vi "DPOAE I-O.vi"(0 "State in":T4) -> (4 "State out":T4)   [LabVIEW 2020]
uses:
  CFTS VIs/CFTS-Experiment State.ctl
  Typedefs/DP-Queue Data.ctl
  Typedefs/DP-Parameters.ctl
  Typedefs/DP-Stimulus Params.ctl
  Typedefs/DP-Response Params.ctl
  epl-vi-lib/Utility VIs/File IO VIs/Configuration File Wrapper VIs/Config-Write Key (string).vi
panel:
  in  "Probe Mic Gain (dB)":dbl
  in  "Save raw data?":bool=TRUE
  out "User":string
  out "Run #":u16=14
  out "ID #":u16=1
  in  "Avg specs":T1={"# Time avgs "=8, "# Spectrum avgs"=4}
  in  "Stimulus":T2={"Ear"=enum."Right", "f2 freqs (kHz)"="5.6;8.0;11.3;16;22.6;32;", "Start (dB)"=20.0, "Stop (dB)"=70.0, "Step (dB)"=10.0, "Mode"=enum."L1 = L2 + 10 dB"}
  out "result":T3
  out "Path":path
  in  "Start":bool
  in  "Stop":bool
  out "Error":bool
  out "Freqs":cluster{"f1":dbl, "f2":dbl, "2f1-f2":dbl}={"f1"=9419.759114583332, "f2"=11291.50390625, "2f1-f2"=7548.014322916664} {"2f1-f2" format="%.3f"; "f1" format="%.3f"; "f2" format="%.3f"}
  out "DP window":cluster{i32, "df (Hz)":dbl, dbl[]}(graph)={0, "df (Hz)"=0.02, []}
  out "I-O Plot":cluster{cluster{dbl, dbl}[]}[](graph)
  in  "Notes":string
  out "Full Spectrum":cluster{i32, "Freq Resolution":dbl, dbl[]}(graph)={0, "Freq Resolution"=20.345052083333332, []}
  in  "RETURN":bool
  # "Stimulus"
  # "Averaging"
  # "Response"
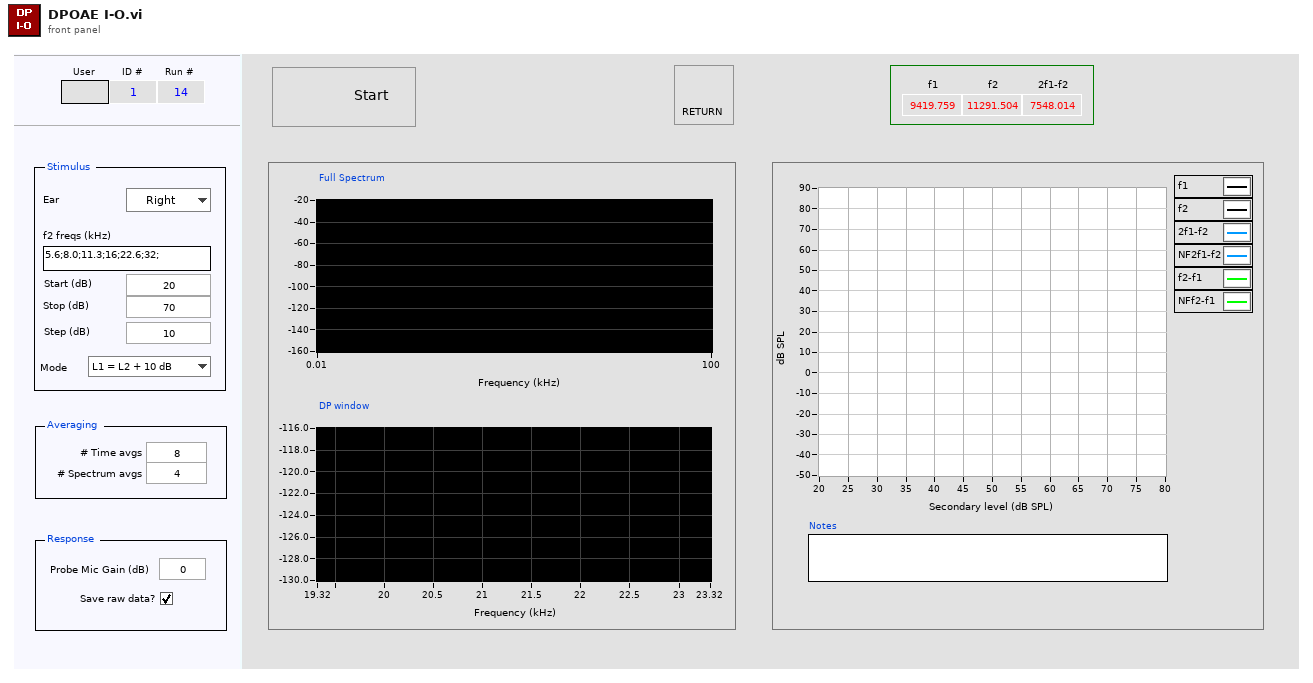
[diagram p1: front panel]
types:
  T1 = cluster{"# Time avgs ":i32, "# Spectrum avgs":i32}
  T2 = cluster{"Ear":enum16{"Right", "Left"}, "f2 freqs (kHz)":string, "Start (dB)":dbl, "Stop (dB)":dbl, "Step (dB)":dbl, "Mode":enum16{"L1 = L2", "L1 = L2 + 10 dB"}}
  T3 = cluster{"file":path, "aborted":bool, "error":errorcluster}
  T4 = typedef "CFTS-Experiment State.ctl" = cluster{"Experimenter":string, "Number":u32, "Right":string, "Left":string, "Data Folder":path, "Version":string, "End Exposure Time":dbl, "Exposure Duration":string, "Run #":cluster{"CAP":i32, "ABR":i32, "DP":i32, "VsEP":i32, "SFOAE":i32}}
  T5 = typedef "DP-Queue Data.ctl" = cluster{"action":string, "path":path, "Acoustic system":string, "Parameters":T6}
  T6 = typedef "DP-Parameters.ctl" = cluster{"Stimulus":T7, "Response":T8}
  T7 = typedef "DP-Stimulus Params.ctl" = cluster{"Ear":enum16{"Right", "Left"}, "f2 freqs (kHz)":string, "Start (dB)":dbl, "Stop (dB)":dbl, "Step (dB)":dbl, "Mode":enum16{"L1 = L2", "L1 = L2 + 10 dB"}, "override recal":bool, "Sampling Rate (Hz)":dbl, "Frame (ms)":dbl}
  T8 = typedef "DP-Response Params.ctl" = cluster{"Time avgs":i32, "Freq avgs":i32, "Mic gain (dB)":dbl, "Save raw":bool}
  T9 = enum8{"Enabled", "Disabled", "Disabled and Grayed Out"}
  T10 = typedef "DP-Runtime State.ctl" = cluster{"#spectra avgs":i32[], "#time avgs":i32[], "dt (ms)":dbl, "df (kHz)":dbl, "pts/frame":i32, "Save raw?":bool, "Data File":path, "Sampling rate (Hz)":dbl, "Probe Tube Sensitivity":cluster{"Frequency":dbl[], "Mag":dbl[], "Phase":dbl[]}, "Mic gain (dB)":dbl, "frames/buffer":i32, "pts/buffer":i32, "speakers":string[], "mic":string}
  T11 = typedef "DP-Freqs.ctl" = cluster{"f1":dbl, "f2":dbl, "2f1-f2":dbl}
  T12 = typedef "DP-Level Series Info.ctl" = cluster{"freq":dbl[], "atten":dbl[][], "ntime":i32[], "nfreq":i32[], "raw file":path, "flip":bool}
  T13 = cluster{"Data File":path, "aborted":bool, "error out":errorcluster}
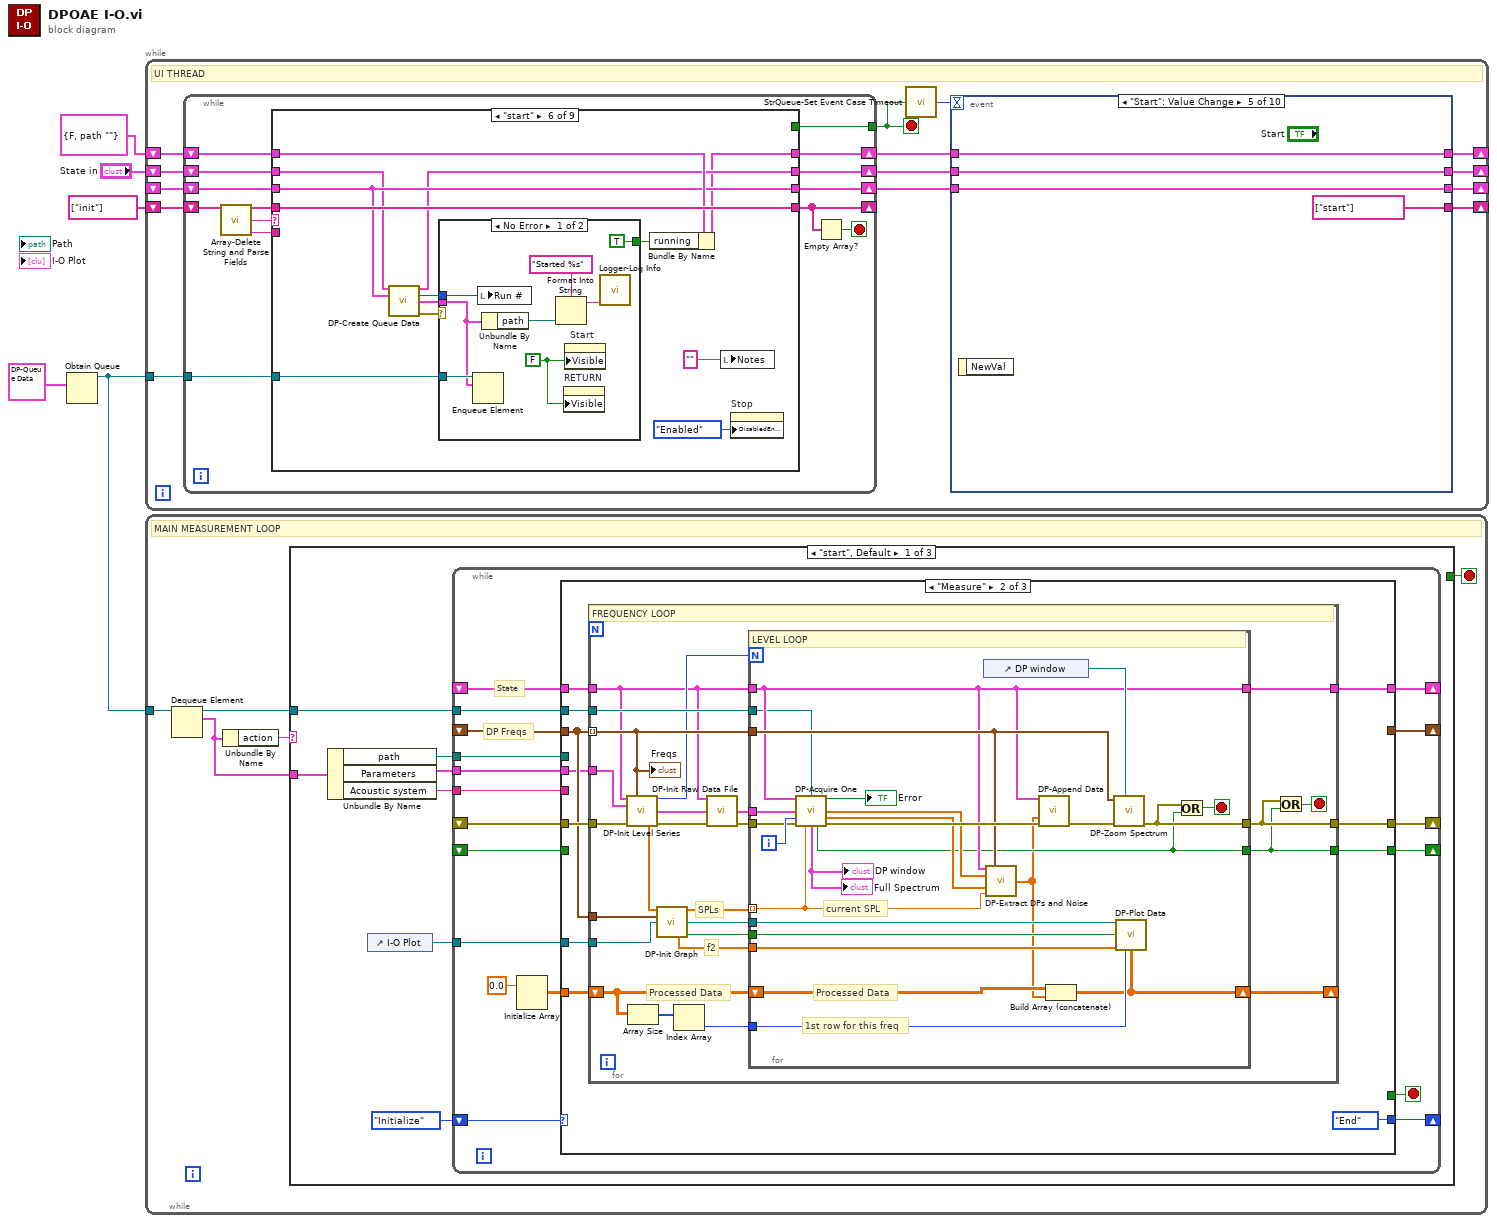
[diagram p0: block diagram]
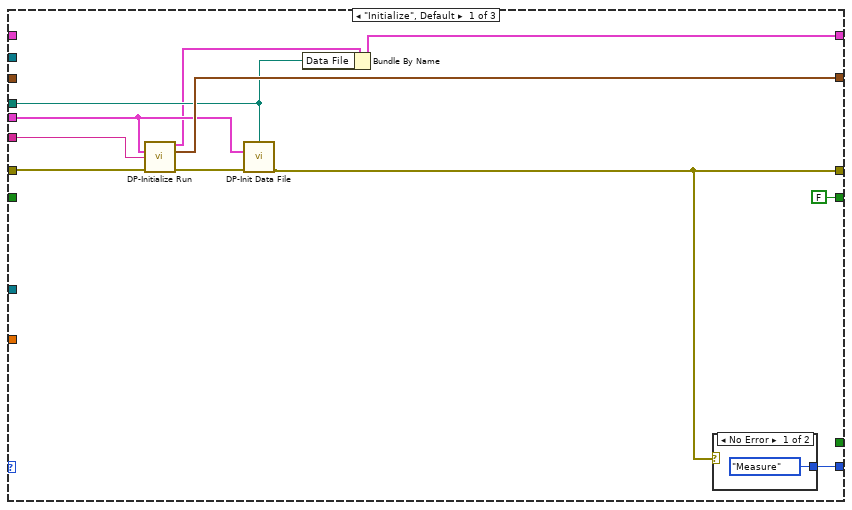
[diagram p2: hidden frame]
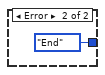
[diagram p3: hidden frame]
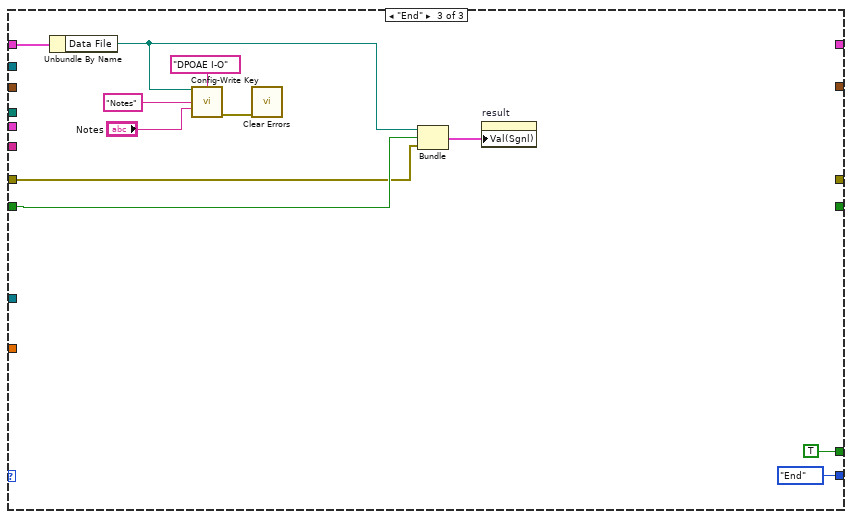
[diagram p4: hidden frame]
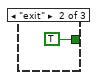
[diagram p5: hidden frame]
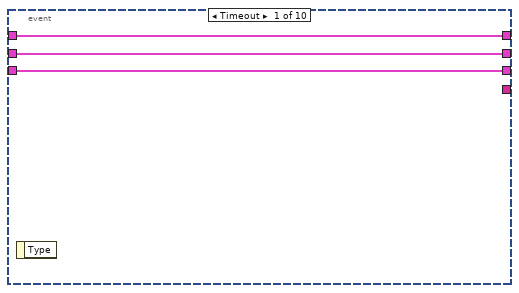
[diagram p7: hidden frame]
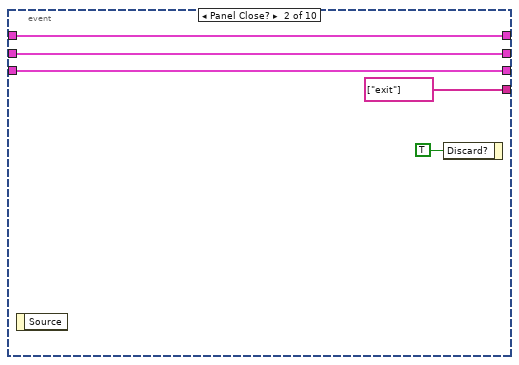
[diagram p8: hidden frame]
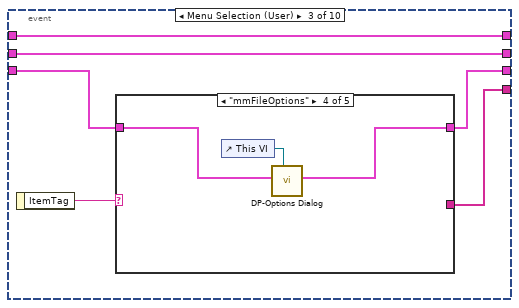
[diagram p9: hidden frame]
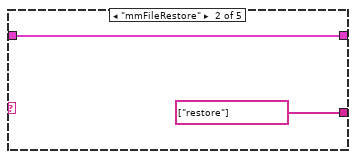
[diagram p11: hidden frame]
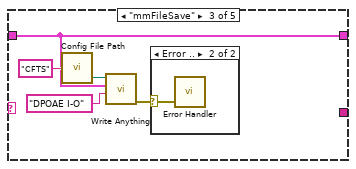
[diagram p12: hidden frame]
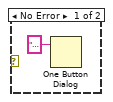
[diagram p13: hidden frame]
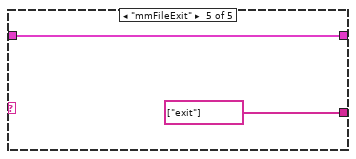
[diagram p14: hidden frame]
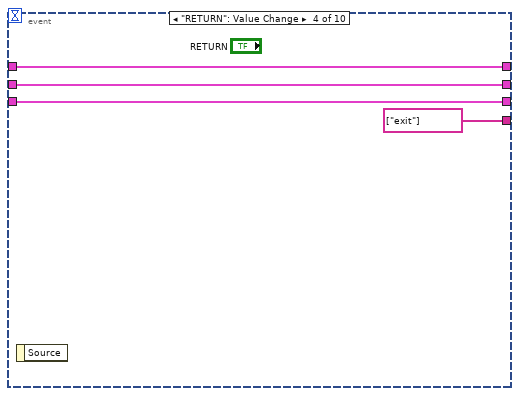
[diagram p15: hidden frame]
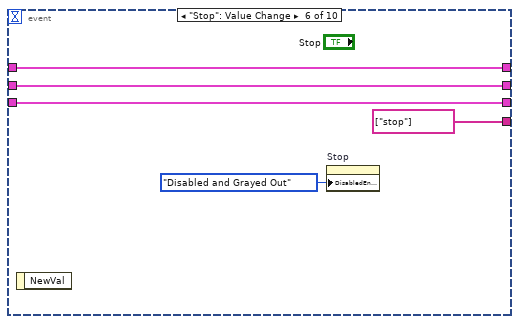
[diagram p16: hidden frame]
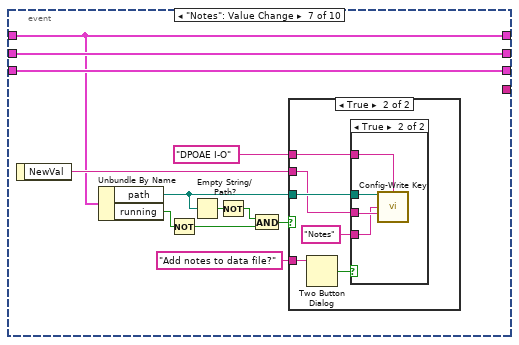
[diagram p17: hidden frame]
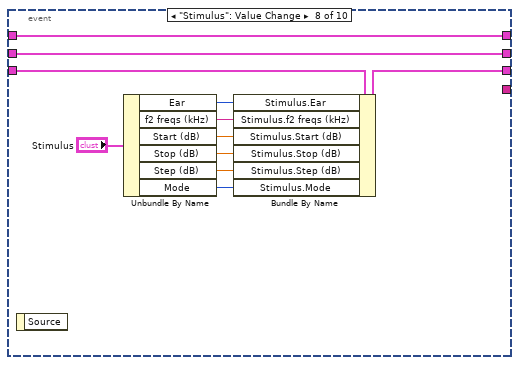
[diagram p20: hidden frame]
diagram:
  n1 = Obtain Queue(element data type=T5 {"action"="", "path"=path "", "Acoustic system"="", "Parameters"={"Stimulus"={"Ear"=enum."Right", "f2 freqs (kHz)"="", "Start (dB)"=0.0, "Stop (dB)"=0.0, "Step (dB)"=0.0, "Mode"=enum."L1 = L2", "override recal"=FALSE, "Sampling Rate (Hz)"=0.0, "Frame (ms)"=0.0}, "Response"={"Time avgs"=0, "Freq avgs"=0, "Mic gain (dB)"=0.0, "Save raw"=FALSE}}} ("data")) -> (queue out=w2:refnum<queue>)  [unwired: 4 in, 2 out]
  n2 = while {
    tunnel: w2 -> [w16]
    shift-right: [w14] -> _
    shift-left: string[] ["init"] -> [w15]
    shift-right: [w12] -> _
    shift-left: cluster{"running":bool, "path":path} {"running"=FALSE, "path"=path ""} -> [w13]
    shift-right: [w10] -> _
    shift-left: "State in" -> [w17]
    shift-right: [w8] -> _
    shift-left: _ -> [w6]
    stop <- w18 stop-if-true
    # "UI THREAD"
    n3 = while {
      shift-right: [w146] -> _
      shift-left: w15 -> [w143]
      tunnel: [w144] -> w18
      tunnel: w16 -> [w139]
      shift-right: [w137] -> w11
      shift-left: w13 -> [w138]
      shift-right: [w136] -> w9
      shift-left: w17 -> [w140]
      shift-right: [w135] -> w7
      shift-left: w6 -> [w134]
      stop <- w145 stop-if-true
      n4 = call "Array-Delete String and Parse Fields.vi"("Array in"=w143) -> ("Array out"=w142:string[], "Field 1"=w141:string, "Field 2"=w133:string)  [unwired: 10 in, 2 out]
      n5 = case shown="\"start\"" w141 {
        tunnel: w142 -> [w150 w159 _ w174 w192 w205 w223 w226 w257]
        tunnel: [w150 w159 string[] ["restore"] ("Array out") w170 w192 w205 w223 w225 w257] -> w146
        tunnel: [_ TRUE _ _ _ _ _ _ _] -> w144
        tunnel: w140 -> [w148 w156 w165 w172 w190 w197 w221 w229 w254]
        tunnel: w139 -> [_ w152 _ _ _ w201 w216 _ _]
        tunnel: w138 -> [w149 w157 w163 w173 w191 w202 w222 w230 w256]
        tunnel: [w149 w157 w163 w173 w191 w194 w222 w230 w256] -> w137
        tunnel: [w148 w156 w165 w172 w190 w196 w221 w224 w254] -> w136
        tunnel: [w147 w155 w161 w171 w181 w198 w220 w235 w255] -> w135
        tunnel: w134 -> [w147 w155 w161 _ w181 w198 w220 w235 w255]
        tunnel: w133 -> [_ _ _ _ _ _ _ w227 _]
        frame "", Default {
        }
        frame "exit" {
          n6 = Bundle By Name(cluster=T5 {"action"="", "path"=path "", "Acoustic system"="", "Parameters"={"Stimulus"={"Ear"=enum."Right", "f2 freqs (kHz)"="", "Start (dB)"=0.0, "Stop (dB)"=0.0, "Step (dB)"=0.0, "Mode"=enum."L1 = L2", "override recal"=FALSE, "Sampling Rate (Hz)"=0.0, "Frame (ms)"=0.0}, "Response"={"Time avgs"=0, "Freq avgs"=0, "Mic gain (dB)"=0.0, "Save raw"=FALSE}}} ("data"), "action"="exit") -> (w151:T5)
          n7 = Enqueue Element(queue=w152, element=w151) -> ()  [unwired: 2 in, 3 out]
          "State out" <- w156
        }
        frame "init" {
          w164 = TRUE
          n8 = Unbundle By Name(w165) -> ("Experimenter"=→"User":string, "Number"=→"ID #":u32, "Run #.DP"=→"Run #":i32)
          n9 = property on="RETURN" class="Bool"("Visible"=w164) -> ()  [unwired: 2 in, 2 out]
          n10 = property on="Start" class="Bool"("Visible"=w164) -> ()  [unwired: 2 in, 2 out]
          n11 = local write "Error"(FALSE ("Error")) -> ()
        }
        frame "restore" {
          n12 = call "DP-Restore Defaults.vi"() -> ("Parameters"=w171:T6)  [unwired: 14 in, 1 out]
          n13 = Build Array (concatenate)(w174, "show params") -> (w170:string[])
        }
        frame "show params" {
          n14 = Unbundle By Name(w181) -> ("Stimulus.Ear"=w188:enum16{"Right", "Left"}, "Stimulus.f2 freqs (kHz)"=w187:string, "Stimulus.Start (dB)"=w186:dbl, "Stimulus.Stop (dB)"=w185:dbl, "Stimulus.Step (dB)"=w184:dbl, "Stimulus.Mode"=w183:enum16{"L1 = L2", "L1 = L2 + 10 dB"})
          n15 = Unbundle By Name(w181) -> ("Response.Time avgs"=w179:i32, "Response.Freq avgs"=w178:i32, "Response.Mic gain (dB)"=w176:dbl, "Response.Save raw"=w175:bool)
          n16 = local read "Stimulus"() -> (w189:T2)
          n17 = local write "Probe Mic Gain (dB)"(w176) -> ()
          n18 = local write "Save raw data?"(w175) -> ()
          n19 = Bundle By Name(cluster=w189, "Ear"=w188, "f2 freqs (kHz)"=w187, "Start (dB)"=w186, "Stop (dB)"=w185, "Step (dB)"=w184, "Mode"=w183) -> (w182:T2)
          n20 = local read "Avg specs"() -> (w180:T1)
          n21 = Bundle By Name(cluster=w180, "# Time avgs"=w179, "# Spectrum avgs"=w178) -> (w177:T1)
          n22 = local write "Stimulus"(w182) -> ()
          n23 = local write "Avg specs"(w177) -> ()
        }
        frame "start" {
          n24 = call "DP-Create Queue Data.vi"("State in"=w197, "Parameters"=w198) -> ("State out"=w196:T4, "run"=w195:i32, "data"=w200:T5, "error out"=w199:errorcluster)  [unwired: 10 in]
          n25 = case shown="No Error" w199 {
            selector: w199 -> [_ w215]
            tunnel: w201 -> [w213 _]
            tunnel: w200 -> [w209 _]
            tunnel: w195 -> [w211 _]
            tunnel: [TRUE _] -> w193
            frame No Error {
              w212 = FALSE
              n26 = Enqueue Element(queue=w213, element=w209) -> ()  [unwired: 2 in, 3 out]
              n27 = local write "Run #"(w211) -> ()
              n28 = Unbundle By Name(w209) -> ("path"=w208:path)
              n29 = Format Into String(format string="Started %s", w208) -> (resulting string=w206:string)  [unwired: 2 in, 1 out]
              n30 = property on="RETURN" class="Bool"("Visible"=w212) -> ()  [unwired: 2 in, 2 out]
              n31 = property on="Start" class="Bool"("Visible"=w212) -> ()  [unwired: 2 in, 2 out]
              n32 = call "Logger-Log Info.vi"("Message"=w206) -> ()  [unwired: 14 in, 1 out]
            }
            frame Error {
              n33 = call "Logger-Check and Log Error.vi"("error in (no error)"=w215) -> ("error out"=w214:errorcluster)  [unwired: 14 in]
              n34 = call "Error Handler.vi"("error in (no error)"=w214) -> ()  [unwired: 12 in, 3 out]
            }
          }
          n35 = Bundle By Name(cluster=w202, "running"=w193) -> (w194:cluster{"running":bool, "path":path})
          n36 = local write "Notes"("" ("Notes")) -> ()
          n37 = property on="Stop" class="Bool"("DisabledEnum"=T9."Enabled" ("Disabled")) -> ()  [unwired: 2 in, 2 out]
        }
        frame "stop" {
          n38 = Bundle By Name(cluster=T5 {"action"="", "path"=path "", "Acoustic system"="", "Parameters"={"Stimulus"={"Ear"=enum."Right", "f2 freqs (kHz)"="", "Start (dB)"=0.0, "Stop (dB)"=0.0, "Step (dB)"=0.0, "Mode"=enum."L1 = L2", "override recal"=FALSE, "Sampling Rate (Hz)"=0.0, "Frame (ms)"=0.0}, "Response"={"Time avgs"=0, "Freq avgs"=0, "Mic gain (dB)"=0.0, "Save raw"=FALSE}}} ("data"), "action"="stop") -> (w217:T5)
          n39 = Enqueue Element(queue=w216, element=w217) -> ()  [unwired: 2 in, 3 out]
        }
        frame "dispose" {
          n40 = Unbundle By Name(w229) -> ("Data Folder"=w228:path)
          n41 = Two Button Dialog(message="Data collection was aborted.\nSave data?", 1:"No" ("F button name (\"Cancel\")"), 2:"Yes" ("T button name (\"OK\")")) -> (T button?=w234:bool)
          n42 = case shown="False" w234 {
            tunnel: w226 -> [_ w251]
            tunnel: [_ w251] -> w225
            tunnel: w227 -> [w248 _]
            tunnel: w228 -> [w249 _]
            tunnel: w229 -> [w241 w250]
            tunnel: w230 -> [w244 w252]
            tunnel: [w243 w252] -> _
            tunnel: [w237 w250] -> w224
            frame False {
              n43 = Unbundle By Name(w241) -> ("Run #.DP"=w239:i32)
              n44 = Concatenate Strings(w248, ".*" ("string")) -> (w246:string)
              n45 = Decrement(x=w239) -> (x-1=w238:i32)
              n46 = Bundle By Name(cluster=w241, "Run #.DP"=w238) -> (w240:T4)
              n47 = call "FileIO-Delete Files.vi"("Folder"=w249, "Pattern"=w246) -> ()  [unwired: 13 in, 1 out]
              n48 = Concatenate Strings("Deleted " ("string"), w246) -> (w236:string)
              n49 = call "CFTS-Write State.vi"("State"=w240) -> ("State thru"=w237:T4)  [unwired: 13 in, 1 out]
              n50 = call "Logger-Log Info.vi"("Message"=w236) -> ()  [unwired: 14 in, 1 out]
              n51 = Bundle By Name(cluster=w244, "path"=path "") -> (w243:cluster{"running":bool, "path":path})
            }
            frame True {
            }
          }
        }
        frame "analysis" {
          n52 = Unbundle By Name(w254) -> ("Data Folder"=w253:path)
          n53 = call "DPOAE Analysis Panel.vi"("Data folder in"=w253) -> ()  [unwired: 11 in]
        }
      }
      n54 = Empty Array?(array=w146) -> (empty?=w145:bool)
    }
    n55 = call "StrQueue-Set Event Case Timeout.vi"("Quit"=w18) -> ("timeout"=w19:i32)  [unwired: 14 in]
    n56 = event shown="[4] \"Start\": Value Change" {
      selector: _ -> [_ _ _ _ _ _ _ _ _ _]
      dyn-events: _ -> [_ _ _ _ _ _ _ _ _ _]
      timeout: w19 -> [_ _ _ _ _ _ _ _ _ _]
      tunnel: [_ string[] ["exit"] w32 string[] ["exit"] string[] ["start"] ("Array out") string[] ["stop"] ("Array out") _ _ _ w107] -> w14
      tunnel: [w22 w25 w31 w51 w56 w61 w62 w94 w103 w106] -> w12
      tunnel: w11 -> [w22 w25 w31 w51 w56 w61 w62 w94 w103 w121]
      tunnel: [w21 w24 w30 w50 w55 w60 w73 w93 w102 w108] -> w10
      tunnel: w9 -> [w21 w24 w30 w50 w55 w60 w73 w93 w102 w108]
      tunnel: [w20 w23 w28 w49 w54 w59 w72 w91 w99 w120] -> w8
      tunnel: w7 -> [w20 w23 w29 w49 w54 w59 w72 w92 w101 w120]
      event Timeout {
        n57 = event-data() -> ()  [unwired: 1 in, 1 out]
      }
      event Panel Close? {
        n58 = event-data() -> ()  [unwired: 1 in, 1 out]
        n59 = event-data("Discard?"=TRUE) -> ()  [unwired: 1 in, 1 out]
      }
      event Menu Selection (User) {
        n60 = event-data() -> ("ItemTag"=w33:string)  [unwired: 1 in]
        n61 = case shown="\"mmFileOptions\"" w33 {
          tunnel: [_ string[] ["restore"] ("Array out") _ _ string[] ["exit"]] -> w32
          tunnel: w29 -> [w34 w35 w37 w45 w47]
          tunnel: [w34 w35 w37 w44 w47] -> w28
          frame Default {
          }
          frame "mmFileRestore" {
          }
          frame "mmFileSave" {
            n62 = call "Config File Path.vi"("AppName"="CFTS") -> ("Default config file name"=w40:path)
            n63 = call "Write Anything.vi"("Section Name (Name of \"Anything\")"="DPOAE I-O" ("Section Name (Name of \"Type of Anything\")"), "Anything"=w37, "Path (dialog)"=w40) -> ("Error Out"=w38:errorcluster)  [unwired: 7 in, 1 out]
            n64 = case shown="Error .." w38 {
              selector: w38 -> [_ w43]
              frame No Error {
                n65 = One Button Dialog(message="Defaults saved.") -> ()  [unwired: 1 in, 1 out]
              }
              frame Error {
                n66 = call "Error Handler.vi"("error in (no error)"=w43) -> ()  [unwired: 12 in, 3 out]
              }
            }
          }
          frame "mmFileOptions" {
            n67 = control-ref of="This VI"() -> (w46:refnum<vi>)
            n68 = call "DP-Options Dialog.vi"("Parent VI"=w46, "Param in"=w45) -> ("Param out"=w44:T6)  [unwired: 8 in, 1 out]
          }
          frame "mmFileExit" {
          }
        }
      }
      event "RETURN": Value Change {
        n69 = event-data() -> ()  [unwired: 1 in, 1 out]
      }
      event "Start": Value Change {
        n70 = event-data() -> ()  [unwired: 1 in, 1 out]
      }
      event "Stop": Value Change {
        n71 = event-data() -> ()  [unwired: 1 in, 1 out]
        n72 = property on="Stop" class="Bool"("DisabledEnum"=T9."Disabled and Grayed Out" ("Disabled")) -> ()  [unwired: 2 in, 2 out]
      }
      event "Notes": Value Change {
        n73 = event-data() -> ("NewVal"=w63:string)  [unwired: 1 in]
        n74 = Unbundle By Name(w62) -> ("path"=w66:path, "running"=w65:bool)
        n75 = Not(x=w65) -> (.not. x?=w70:bool)
        n76 = Empty String/Path?(string/path=w66) -> (empty?=w71:bool)
        n77 = Not(x=w71) -> (.not. x?=w69:bool)
        n78 = And(x=w69, y=w70) -> (x .and. y?=w68:bool)
        n79 = case shown="True" w68 {
          tunnel: w66 -> [_ w79]
          tunnel: w63 -> [_ w78]
          tunnel: "Add notes to data file?" ("message") -> [_ w77]
          tunnel: "DPOAE I-O" -> [_ w74]
          frame False {
          }
          frame True {
            n80 = Two Button Dialog(message=w77) -> (T button?=w76:bool)  [unwired: 2 in]
            n81 = case shown="True" w76 {
              tunnel: w79 -> [_ w83]
              tunnel: w78 -> [_ w82]
              tunnel: "Notes" -> [_ w81]
              tunnel: w74 -> [_ w80]
              frame False {
              }
              frame True {
                n82 = call-poly "Config-Write Key.vi"("configuration file path"=w83, "section"=w80, "key"=w81, "value"=w82) -> ()  [unwired: 9 in, 3 out]
              }
            }
          }
        }
      }
      event "Stimulus": Value Change {
        n83 = event-data() -> ()  [unwired: 1 in, 1 out]
        n84 = Unbundle By Name("Stimulus") -> ("Ear"=w89:enum16{"Right", "Left"}, "f2 freqs (kHz)"=w88:string, "Start (dB)"=w87:dbl, "Stop (dB)"=w86:dbl, "Step (dB)"=w85:dbl, "Mode"=w84:enum16{"L1 = L2", "L1 = L2 + 10 dB"})
        n85 = Bundle By Name(cluster=w92, "Stimulus.Ear"=w89, "Stimulus.f2 freqs (kHz)"=w88, "Stimulus.Start (dB)"=w87, "Stimulus.Stop (dB)"=w86, "Stimulus.Step (dB)"=w85, "Stimulus.Mode"=w84) -> (w91:T6)
      }
      event "Avg specs", "Probe Mic Gain (dB)", "Save raw data?": Value Change {
        n86 = event-data() -> ()  [unwired: 1 in, 1 out]
        n87 = Unbundle By Name("Avg specs") -> ("# Time avgs"=w98:i32, "# Spectrum avgs"=w97:i32)
        n88 = Bundle By Name(cluster=w101, "Response.Time avgs"=w98, "Response.Freq avgs"=w97, "Response.Mic gain (dB)"="Probe Mic Gain (dB)", "Response.Save raw"="Save raw data?") -> (w99:T6)
      }
      event "result": Value Change {
        w119 = TRUE
        n89 = event-data() -> ("NewVal.error"=w111:errorcluster, "NewVal.aborted"=w110:bool, "NewVal.file"=w109:path)  [unwired: 1 in]
        n90 = property on="RETURN" class="Bool"("Visible"=w119) -> ()  [unwired: 2 in, 2 out]
        n91 = property on="Start" class="Bool"("Visible"=w119) -> ()  [unwired: 2 in, 2 out]
        n92 = call "Error Handler.vi"("error in (no error)"=w111) -> ("error?"=w113:bool)  [unwired: 12 in, 2 out]
        n93 = call <vilib>:"Get File Extension.vi"("file"=w109) -> ("filename without extension"=w116:string, "dup file"=w105:path)  [unwired: 6 in, 3 out]
        n94 = Unbundle By Name(w111) -> ("status"=w117:bool, "code"=w118:i32)
        n95 = Or(x=w113, y=w110) -> (x .or. y?=w114:bool)
        n96 = case shown="True" w114 {
          tunnel: [_ w128] -> w115
          tunnel: w116 -> [_ w125]
          tunnel: w108 -> [_ _]
          tunnel: w117 -> [_ w124]
          tunnel: w118 -> [_ w123]
          frame False {
            n97 = call "Logger-Log Info.vi"("Message"="Finished" ("message")) -> ()  [unwired: 14 in, 1 out]
          }
          frame True {
            n98 = case shown="False" w124 {
              tunnel: w123 -> [_ w132]
              frame False {
                n99 = call "Logger-Log Info.vi"("Message"="Aborted") -> ()  [unwired: 14 in, 1 out]
              }
              frame True {
                n100 = Format Into String(format string="Error: %d", w132) -> (resulting string=w130:string)  [unwired: 2 in, 1 out]
                n101 = call "Logger-Log Error.vi"("Message"=w130) -> ()  [unwired: 14 in, 1 out]
              }
            }
            n102 = Format Into String(format string="dispose:%s", w125) -> (resulting string=w126:string)  [unwired: 2 in, 1 out]
            n103 = Build Array(w126) -> (w128:string[])
          }
        }
        n104 = Bundle By Name(cluster=w121, "path"=w105, "running"=FALSE) -> (w106:cluster{"running":bool, "path":path})
        n105 = Build Array (concatenate)("analysis", w115) -> (w107:string[])
      }
    }
  }
  n106 = while {
    tunnel: w2 -> [w262]
    stop <- w260 stop-if-true
    # "MAIN MEASUREMENT LOOP"
    n107 = Dequeue Element(queue=w262) -> (queue out=w258:refnum<queue>, element=w259:T5)  [unwired: 2 in, 2 out]
    n108 = Unbundle By Name(w259) -> ("action"=w261:string)
    n109 = case shown="\"start\", Default" w261 {
      tunnel: [_ TRUE _] -> w260
      tunnel: w259 -> [w269 _ _]
      tunnel: w258 -> [w268 _ _]
      frame "start", Default {
        n110 = Unbundle By Name(w269) -> ("path"=w264:path, "Parameters"=w266:T6, "Acoustic system"=w265:string)
        n111 = control-ref of="I-O Plot"() -> (w263:refnum<vi>)
        n112 = while {
          shift-right: [w286] -> _
          shift-left: _ -> [w287]
          shift-right: [w281] -> _
          shift-left: enum16{"Initialize", "Measure", "End"}."Initialize" -> [w285]
          shift-right: [w282] -> _
          shift-left: _ -> [w283]
          shift-right: [w280] -> _
          shift-left: _ -> [w279]
          tunnel: w266 -> [w276]
          tunnel: w265 -> [w270]
          tunnel: w264 -> [w275]
          tunnel: w263 -> [w274]
          tunnel: w268 -> [w273]
          shift-right: [w272] -> _
          shift-left: _ -> [w271]
          stop <- w284 stop-if-true
          # "State"
          # "DP Freqs"
          n113 = Initialize Array(0.0) -> (w277:dbl[][])  [unwired: 2 in]
          n114 = case shown="\"Measure\"" w285 {
            tunnel: w287 -> [w296 w311 w367]
            tunnel: [w295 w310 _] -> w286
            tunnel: [_ _ TRUE] -> w284
            tunnel: w283 -> [_ w308 w369]
            tunnel: [w294 w306 _] -> w282
            tunnel: [w297 enum16{"Initialize", "Measure", "End"}."End" enum16{"Initialize", "Measure", "End"}."End"] -> w281
            tunnel: [w298 _ _] -> w280
            tunnel: w279 -> [_ w305 _]
            tunnel: w277 -> [_ w309 _]
            tunnel: w276 -> [w293 w304 _]
            tunnel: w270 -> [w292 _ _]
            tunnel: w275 -> [w291 _ _]
            tunnel: w274 -> [_ w303 _]
            tunnel: w273 -> [_ w302 _]
            tunnel: [FALSE ("aborted") w301 _] -> w272
            tunnel: w271 -> [_ _ w368]
            frame "Initialize", Default {
              n115 = call "DP-Initialize Run.vi"("Parameters"=w293, "acoustic system"=w292, "error in (no error)"=w296) -> ("State"=w289:T10, "DP Freqs"=w298:T11[], "error out"=w288:errorcluster)  [unwired: 10 in]
              n116 = call "DP-Init Data File.vi"("Path"=w291, "Parameters"=w293, "error in (no error)"=w288) -> ("error out"=w295:errorcluster)  [unwired: 12 in]
              n117 = Bundle By Name(cluster=w289, "Data File"=w291) -> (w294:T10)
              n118 = case shown="No Error" w295 {
                tunnel: [enum16{"Initialize", "Measure", "End"}."Measure" enum16{"Initialize", "Measure", "End"}."End"] -> w297
                frame No Error {
                }
                frame Error {
                }
              }
            }
            frame "Measure" {
              n119 = for {
                shift-right: [w332] -> _
                shift-left: w309 -> [w336]
                tunnel: w311 -> [w333]
                tunnel: [w321] -> w310
                tunnel: w305 -> [w319] mode=indexing
                tunnel: w308 -> [w313]
                tunnel: [w331] -> w306
                tunnel: w305 -> [w328]
                tunnel: w304 -> [w323]
                tunnel: w303 -> [w324]
                tunnel: w302 -> [w322]
                tunnel: [w312] -> w301
                stop <- w320 stop-if-true
                # "f2"
                # "SPLs"
                # "Processed Data"
                # "FREQUENCY LOOP"
                n120 = call "DP-Init Level Series.vi"("state"=w313, "DP Freqs"=w319, "Parameters"=w323, "error in (no error)"=w333) -> ("num levels"=w318:i32, "level series"=w316:T12, "Nominal f2 SPL"=w330:dbl[], "error out"=w317:errorcluster)  [unwired: 8 in]
                n121 = Array Size(array=w336) -> (size(s)=w335:i32[])
                n122 = call "DP-Init Graph.vi"("Nominal f2 SPL in"=w330, "DP Freqs"=w328, "XYGraph in"=w324) -> ("Nominal f2 SPL out"=w329:dbl[], "XYGraph out"=w327:refnum<vi>, "f2"=w325:dbl[], "plot vs freq"=w326:bool)  [unwired: 9 in]
                n123 = Index Array(array=w335) -> (element=w334:i32)  [unwired: 1 in]
                n124 = call "DP-Init Raw Data File.vi"("state"=w313, "level series in"=w316, "error in (no error)"=w317) -> ("level series out"=w315:T12, "error out"=w314:errorcluster)  [unwired: 11 in]
                n125 = for {
                  N: w318 -> [_]
                  tunnel: w329 -> [w337] mode=indexing
                  shift-right: [w351] -> w332
                  shift-left: w336 -> [w360]
                  tunnel: w334 -> [w353]
                  tunnel: w314 -> [w340]
                  tunnel: [w343] -> w321
                  tunnel: w313 -> [w348]
                  tunnel: w319 -> [w349]
                  tunnel: [w348] -> w331
                  tunnel: [w342] -> w312
                  tunnel: w327 -> [w355]
                  tunnel: w326 -> [w354]
                  tunnel: w325 -> [w352]
                  tunnel: w322 -> [w346]
                  tunnel: w315 -> [w341]
                  i -> [w350]
                  stop <- w344 stop-if-true
                  # "current SPL"
                  # "1st row for this freq"
                  # "Processed Data"
                  # "LEVEL LOOP"
                  n126 = call "DP-Acquire One.vi"("State"=w348, "queue"=w346, "level series"=w341, "iLevel"=w350, "error in (no error)"=w340, "L2"=w337) -> ("Error?"=→"Error":bool, "Magnitude"=w358:dbl[], "Phase"=w347:dbl[], "waveform"=→"Full Spectrum" →"DP window":cluster{i32, "dx":dbl, "Array":dbl[]}, "aborted"=w342:bool, "error out"=w359:errorcluster)  [unwired: 4 in]
                  n127 = control-ref of="DP window"() -> (w357:refnum<vi>)
                  n128 = call "DP-Extract DPs and Noise.vi"("state"=w348, "DP Freqs"=w349, "Mag"=w358, "Phase"=w347, "SPL"=w337) -> ("Output Array"=w338:dbl[])  [unwired: 10 in]
                  n129 = call "DP-Append Data.vi"("DataAcq"=w348, "Processed data"=w338, "error in (no error)"=w359) -> ("error out"=w339:errorcluster)  [unwired: 12 in]
                  n130 = Build Array (concatenate)(w360, w338) -> (w351:dbl[][])
                  n131 = call "DP-Zoom Spectrum.vi"("DP window"=w357, "error in (no error)"=w339, "DP Freqs"=w349) -> ("error out"=w343:errorcluster)  [unwired: 8 in]
                  n132 = call "DP-Plot Data.vi"("XYGraph"=w355, "vs Freq"=w354, "f2"=w352, "1st row current freq"=w353, "Input Array (4xn)"=w351) -> ()  [unwired: 11 in]
                  n133 = Or(x=w343, y=w342) -> (x .or. y?=w344:bool)
                }
                n134 = Or(x=w321, y=w312) -> (x .or. y?=w320:bool)
                "Freqs" <- w319
              }
            }
            frame "End" {
              n135 = Unbundle By Name(w369) -> ("Data File"=w363:path)
              n136 = call-poly "Config-Write Key.vi"("configuration file path"=w363, "section"="DPOAE I-O", "key"="Notes", "value"="Notes") -> ("error out"=w361:errorcluster)  [unwired: 9 in, 2 out]
              n137 = call <vilib>:"Clear Errors.vi"("error in (no error)"=w361) -> ()  [unwired: 5 in, 2 out]
              n138 = Bundle("Data File"=w363, "aborted"=w368, "error out"=w367) -> (w362:T13)  [unwired: 1 in]
              n139 = property on="result" class="Clust (strict)"("Val(Sgnl)"=w362) -> ()  [unwired: 2 in, 2 out]
            }
          }
        }
      }
      frame "exit" {
      }
      frame "stop" {
      }
    }
  }
